vi "AI Driver Initialize Channel.vi"(8 "错误输入（无错误）":errorcluster, 9 "Physical Channel":string, 10 "Channel Ref":T2 format="%.0x", 11 "Task in":refnum<k21>) -> (0 "错误输出":errorcluster, 2 "Scale":T1, 3 "Task out":refnum<k21>)   [LabVIEW 2013]
uses:
  <vilib>/K2Labs/HiLab API/Custom Device API/Controls/Custom Device Item Reference.ctl
  Controls/AI Scale.ctl
  MeasurementType.ctl
  AI Terminal Configuration.ctl
  <vilib>/DAQmx/create/channels.llb/DAQmx Create Channel (AI-Voltage-Basic).vi
  <vilib>/DAQmx/create/channels.llb/DAQmx Create Channel (AI-Current-Basic).vi
  <vilib>/K2Labs/HiLab API/Custom Device API/Configuration/Item Properties/Get Item Property/Get Item Property.xnode
  <vilib>/K2Labs/HiLab API/Custom Device API/Custom Device API Library.lvlib
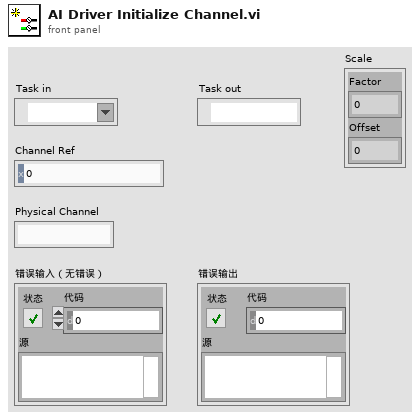
[diagram p1: front panel]
types:
  T1 = typedef "AI Scale.ctl" = cluster{"Factor":dbl, "Offset":dbl}
  T2 = typedef "Custom Device API Library.lvlib/Custom Device Item Reference.ctl" = u64
  T3 = typedef "AI Terminal Configuration.ctl" = enum16{"默认", "RSE", "NRSE", "差分", "伪差分"}
  T4 = typedef "MeasurementType.ctl" = enum16{"Voltage", "Current", "More:Voltage:Custom with Excitation", "More:Current:Custom with Excitation", "Frequency", "Period", "Resistance", "Temperature:Thermocouple", "Temperature:Thermistor", "Temperature:RTD", "Temperature:Built-in Sensor", "Strain Gage"}
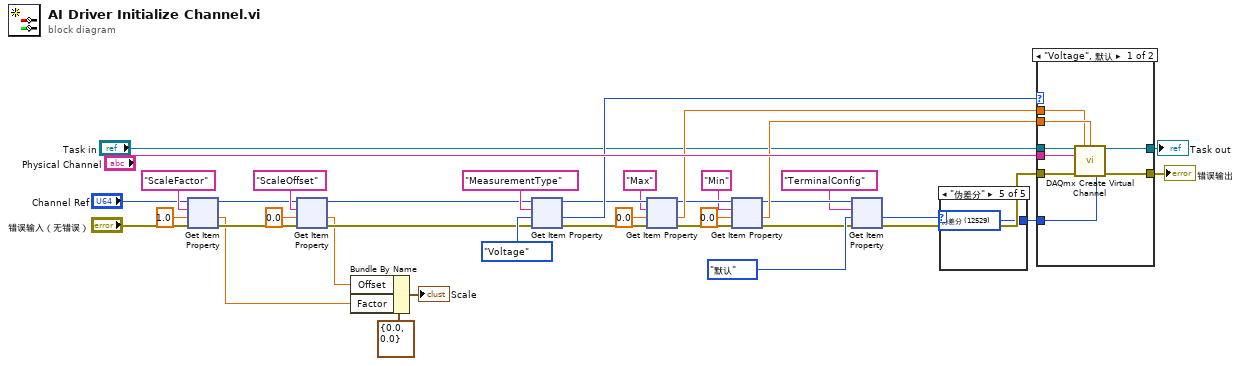
[diagram p0: block diagram]
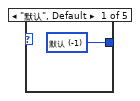
[diagram p2: hidden frame]
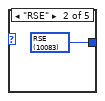
[diagram p3: hidden frame]
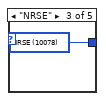
[diagram p4: hidden frame]
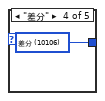
[diagram p5: hidden frame]
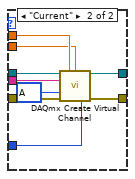
[diagram p6: hidden frame]
diagram:
  n1 = xnode "Get Item Property"("Item Ref in"="Channel Ref", "Property Name"="ScaleFactor", "Default Value"=1.0, "error in (no error)"="错误输入（无错误）") -> ("Item Ref out"=w10:T2, "Value"=w3:dbl, "error out"=w9:errorcluster)  [unwired: 1 out]
  n2 = xnode "Get Item Property"("Item Ref in"=w10, "Property Name"="ScaleOffset", "Default Value"=0.0, "error in (no error)"=w9) -> ("Item Ref out"=w6:T2, "Value"=w2:dbl, "error out"=w5:errorcluster)  [unwired: 1 out]
  n3 = Bundle By Name(cluster=T1 {"Factor"=0.0, "Offset"=0.0} ("Scale"), "Offset"=w2, "Factor"=w3) -> (→"Scale":T1)
  n4 = xnode "Get Item Property"("Item Ref in"=w6, "Property Name"="MeasurementType", "Default Value"=MeasurementType."Voltage" ("MeasurementType"), "error in (no error)"=w5) -> ("Item Ref out"=w30:T2, "Value"=w33:T4, "error out"=w31:errorcluster)  [unwired: 1 out]
  n5 = xnode "Get Item Property"("Item Ref in"=w30, "Property Name"="Max", "Default Value"=0.0, "error in (no error)"=w31) -> ("Item Ref out"=w29:T2, "Value"=w34:dbl, "error out"=w28:errorcluster)  [unwired: 1 out]
  n6 = xnode "Get Item Property"("Item Ref in"=w29, "Property Name"="Min", "Default Value"=0.0, "error in (no error)"=w28) -> ("Item Ref out"=w26:T2, "Value"=w35:dbl, "error out"=w27:errorcluster)  [unwired: 1 out]
  n7 = xnode "Get Item Property"("Item Ref in"=w26, "Property Name"="TerminalConfig", "Default Value"=AI_Terminal_Configuration."默认" ("Terminal Configuration"), "error in (no error)"=w27) -> ("Value"=w15:T3, "error out"=w32:errorcluster)  [unwired: 2 out]
  n8 = case shown="\"伪差分\"" w15 {
    tunnel: [w39 w40 w41 w42 w43] -> w38
    frame "默认", Default {
      w39 = -1 items=["默认"=-1, "RSE"=10083, "NRSE"=10078, "差分"=10106, "伪差分"=12529] ("input terminal configuration")
    }
    frame "RSE" {
      w40 = 10083 items=["默认"=-1, "RSE"=10083, "NRSE"=10078, "差分"=10106, "伪差分"=12529] ("input terminal configuration")
    }
    frame "NRSE" {
      w41 = 10078 items=["默认"=-1, "RSE"=10083, "NRSE"=10078, "差分"=10106, "伪差分"=12529] ("input terminal configuration")
    }
    frame "差分" {
      w42 = 10106 items=["默认"=-1, "RSE"=10083, "NRSE"=10078, "差分"=10106, "伪差分"=12529] ("input terminal configuration")
    }
    frame "伪差分" {
      w43 = 12529 items=["默认"=-1, "RSE"=10083, "NRSE"=10078, "差分"=10106, "伪差分"=12529] ("input terminal configuration")
    }
  }
  n9 = case shown="\"Voltage\", 默认" w33 {
    tunnel: [w49 w60] -> w18
    tunnel: "Task in" -> [w51 w59]
    tunnel: [w48 w58] -> w20
    tunnel: w32 -> [w50 w57]
    tunnel: w34 -> [w46 w55]
    tunnel: w35 -> [w47 w54]
    tunnel: "Physical Channel" -> [w45 w56]
    tunnel: w38 -> [w44 w52]
    frame "Voltage", Default {
      n10 = call-poly <vilib>:"DAQmx Create Virtual Channel.vi"("task in"=w51, "maximum value"=w46, "minimum value"=w47, "input terminal configuration"=w44, "physical channels"=w45, "error in"=w50) -> ("task out"=w49:refnum<k21>, "error out"=w48:errorcluster)  [unwired: 8 in]
    }
    frame "Current" {
      w53 = 10342 items=["A"=10342, "来自自定义换算"=10065] ("units")
      n11 = call-poly <vilib>:"DAQmx Create Virtual Channel.vi"("task in"=w59, "maximum value"=w55, "minimum value"=w54, "input terminal configuration"=w52, "physical channels"=w56, "units"=w53, "error in"=w57) -> ("task out"=w60:refnum<k21>, "error out"=w58:errorcluster)  [unwired: 7 in]
    }
  }
  "错误输出" <- w20
  "Task out" <- w18
